vi "sacar_datos_Sub.vi"(4 "Dato":string) -> (0 "Dato3":dbl, 1 "Dato2":dbl, 2 "Dato1":dbl)   [LabVIEW 2017]
doc: "De la trama de entrada, calcula los valores de los tres sensores"
panel:
  out "sensor3":string
  out "sensor2":string
  out "sensor1":string
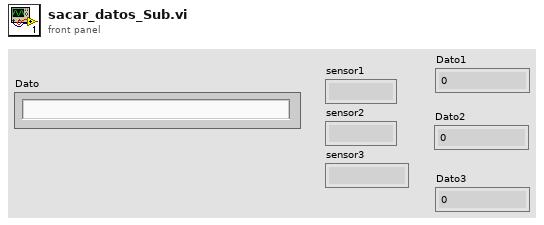
[diagram p1: front panel]
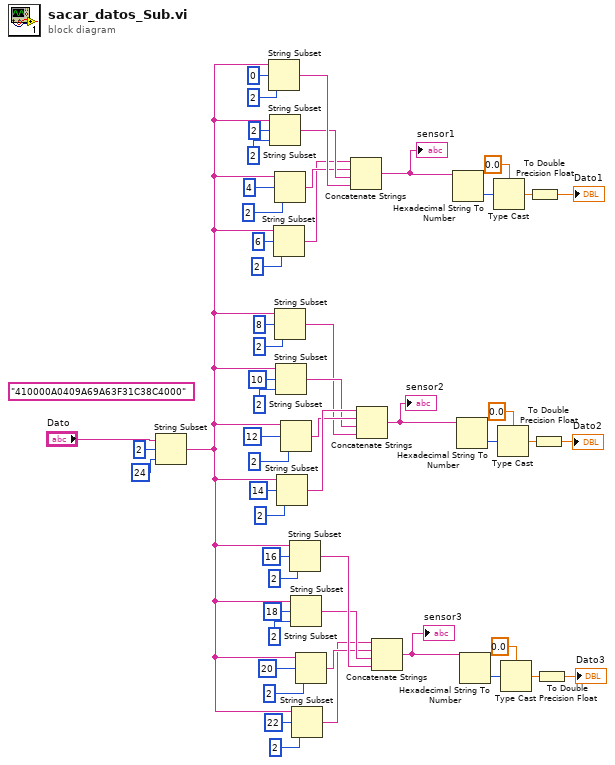
[diagram p0: block diagram]
diagram:
  (unwired) "410000A0409A69A63F31C38C4000"
  n1 = String Subset(string="Dato", offset (0)=2, length (rest)=24 ("length (len. of substring)")) -> (substring=w13:string)
  n2 = String Subset(string=w13, offset (0)=0, length (rest)=2 ("length (rest)")) -> (substring=w46:string)
  n3 = String Subset(string=w13, offset (0)=2, length (rest)=2 ("length (rest)")) -> (substring=w45:string)
  n4 = String Subset(string=w13, offset (0)=6, length (rest)=2 ("length (rest)")) -> (substring=w43:string)
  n5 = String Subset(string=w13, offset (0)=4, length (rest)=2 ("length (rest)")) -> (substring=w44:string)
  n6 = String Subset(string=w13, offset (0)=8, length (rest)=2 ("length (rest)")) -> (substring=w29:string)
  n7 = String Subset(string=w13, offset (0)=10, length (rest)=2 ("length (rest)")) -> (substring=w30:string)
  n8 = String Subset(string=w13, offset (0)=14, length (rest)=2 ("length (rest)")) -> (substring=w32:string)
  n9 = String Subset(string=w13, offset (0)=12, length (rest)=2 ("length (rest)")) -> (substring=w31:string)
  n10 = String Subset(string=w13, offset (0)=16, length (rest)=2 ("length (rest)")) -> (substring=w22:string)
  n11 = String Subset(string=w13, offset (0)=18, length (rest)=2 ("length (rest)")) -> (substring=w21:string)
  n12 = String Subset(string=w13, offset (0)=22, length (rest)=2 ("length (rest)")) -> (substring=w19:string)
  n13 = String Subset(string=w13, offset (0)=20, length (rest)=2 ("length (rest)")) -> (substring=w20:string)
  n14 = Concatenate Strings(w43, w44, w45, w46) -> (w12:string)
  "sensor1" <- w12
  n15 = Concatenate Strings(w32, w31, w30, w29) -> (w8:string)
  "sensor2" <- w8
  n16 = Concatenate Strings(w19, w20, w21, w22) -> (w4:string)
  "sensor3" <- w4
  n17 = Hexadecimal String To Number(string=w12) -> (number=w52:u32)  [unwired: 2 in, 1 out]
  n18 = Hexadecimal String To Number(string=w8) -> (number=w10:u32)  [unwired: 2 in, 1 out]
  n19 = Hexadecimal String To Number(string=w4) -> (number=w6:u32)  [unwired: 2 in, 1 out]
  n20 = Type Cast(type=sgl 0.0 ("Numeric"), x=w52) -> (*(type *) &x=w51:sgl)
  n21 = Type Cast(type=sgl 0.0 ("Numeric"), x=w10) -> (*(type *) &x=w11:sgl)
  n22 = Type Cast(type=sgl 0.0 ("Numeric"), x=w6) -> (*(type *) &x=w5:sgl)
  n23 = To Double Precision Float(number=w51) -> (double precision float=→"Dato1":dbl)
  n24 = To Double Precision Float(number=w11) -> (double precision float=→"Dato2":dbl)
  n25 = To Double Precision Float(number=w5) -> (double precision float=→"Dato3":dbl)
